vi "Export_Clipboard.vi"(7 "Is Copy? (F)":bool, 8 "error in (no error)":errorcluster, 11 "Data in":T1={"Class"={"Ants"=refnum, "Layer"=refnum, "Templates"=refnum, "Icon"=refnum, "Glyph"=refnum, "Settings"=refnum, "Tools"=refnum}, "Ref"={"Add Layer"=refnum, "Remove Layer"=refnum, "Line Text"=[], "Body Text Spec"=refnum, "DNL_Font"=refnum, "glyph path str"=refnum, "templates path str"=refnum, "Arrow Up"=refnum, "Arrow Down"=refnum, "IE VI Ref"=refnum, "Glyphs tree"=refnum, "Templates tree"=refnum, "Layer Icon Text"=refnum, "Layer Template"=refnum, "Clipboard"=refnum, "BW icon in"=refnum, "Color icon in"=refnum, "Layer Clust"=refnum, "Body Text"=refnum, "DNL_Framework Templates"=refnum, "Search Templates"=refnum, "TextMarker"=refnum, "Tab Control"=refnum, "Search Glyphs"=refnum, "Line Color"=refnum, "DNL_Glyphs []"=refnum, "Fill Color"=refnum, "Tools"=refnum, "Glyphs tree"=refnum, "Icon"=refnum, "Preview"=refnum, "Ants"=refnum, "Terminals"=refnum, "menu reference"=refnum, "LayerNames"=[], "GlyphLoadAnimation"=refnum, "TemplateLoadAnimation"=refnum, "refreshGlyphs"=refnum, "refreshTemplates"=refnum}, "Support"={"AntsRect"={"left"=0, "top"=0, "right"=0, "bottom"=0}, "Mouse Move Coords"={"Horizontal"=0, "Vertical"=0}, "Mouse Down Coords"={"Horizontal"=0, "Vertical"=0}, "Temp Coord"={"Horizontal"=0, "Vertical"=0}, "Action"=enum."Default", "Edge Color"=4914962, "Fill Color"=16860, "Mouse Down?"=FALSE, "Draft Mode?"=FALSE, "Temp Icon"=bytes[3102], "CTRL Pressed"=FALSE, "Move Selection?"=FALSE, "AntsRect Orig"={"left"=0, "top"=0, "right"=0, "bottom"=0}, "Text"="", "TM Set?"=FALSE, "Mouse inside icon?"=FALSE, "Tool (old value)"=0, "Pencil Move Color"=0, "Swap Colors?"=FALSE, "Shift pressed?"=FALSE}}) -> (0 "error out":errorcluster, 3 "Data out":T1={"Class"={"Ants"=refnum, "Layer"=refnum, "Templates"=refnum, "Icon"=refnum, "Glyph"=refnum, "Settings"=refnum, "Tools"=refnum}, "Ref"={"Add Layer"=refnum, "Remove Layer"=refnum, "Line Text"=[], "Body Text Spec"=refnum, "DNL_Font"=refnum, "glyph path str"=refnum, "templates path str"=refnum, "Arrow Up"=refnum, "Arrow Down"=refnum, "IE VI Ref"=refnum, "Glyphs tree"=refnum, "Templates tree"=refnum, "Layer Icon Text"=refnum, "Layer Template"=refnum, "Clipboard"=refnum, "BW icon in"=refnum, "Color icon in"=refnum, "Layer Clust"=refnum, "Body Text"=refnum, "DNL_Framework Templates"=refnum, "Search Templates"=refnum, "TextMarker"=refnum, "Tab Control"=refnum, "Search Glyphs"=refnum, "Line Color"=refnum, "DNL_Glyphs []"=refnum, "Fill Color"=refnum, "Tools"=refnum, "Glyphs tree"=refnum, "Icon"=refnum, "Preview"=refnum, "Ants"=refnum, "Terminals"=refnum, "menu reference"=refnum, "LayerNames"=[], "GlyphLoadAnimation"=refnum, "TemplateLoadAnimation"=refnum, "refreshGlyphs"=refnum, "refreshTemplates"=refnum}, "Support"={"AntsRect"={"left"=0, "top"=0, "right"=0, "bottom"=0}, "Mouse Move Coords"={"Horizontal"=0, "Vertical"=0}, "Mouse Down Coords"={"Horizontal"=0, "Vertical"=0}, "Temp Coord"={"Horizontal"=0, "Vertical"=0}, "Action"=enum."Default", "Edge Color"=4914962, "Fill Color"=16860, "Mouse Down?"=FALSE, "Draft Mode?"=FALSE, "Temp Icon"=bytes[3102], "CTRL Pressed"=FALSE, "Move Selection?"=FALSE, "AntsRect Orig"={"left"=0, "top"=0, "right"=0, "bottom"=0}, "Text"="", "TM Set?"=FALSE, "Mouse inside icon?"=FALSE, "Tool (old value)"=0, "Pencil Move Color"=0, "Swap Colors?"=FALSE, "Shift pressed?"=FALSE}})   [LabVIEW 2021]
uses:
  Controls/IE Data.ctl
  Class/Ants/Ants.lvclass
  Class/FakedArray/FakedArray.lvclass
  vi.lib/LabVIEW Icon API/lv_icon/Classes/Icon/Icon.lvclass
  Class/Icon Library/Glyph.lvclass
  Class/Settings/Settings.lvclass
  Class/Tools/Tools Paint.lvclass
  Controls/IE Classes.ctl
  Controls/References Cluster.ctl
  Controls/SupportClass.ctl
  <vilib>/Utility/miscctls.llb/LVPoint32TypeDef.ctl
  Controls/SupportClass_Action.ctl
  vi.lib/LabVIEW Icon API/lv_icon/Controls/IEColor.ctl
  vi.lib/LabVIEW Icon API/lv_icon/Classes/Icon Framework/Icon Framework.lvclass
  C:/projects/labview-icon-editor/source/vi.lib/LabVIEW Icon API/lv_icon/Classes/Layer/Layer.lvclass
  vi.lib/LabVIEW Icon API/lv_icon/lv_icon.lvlib
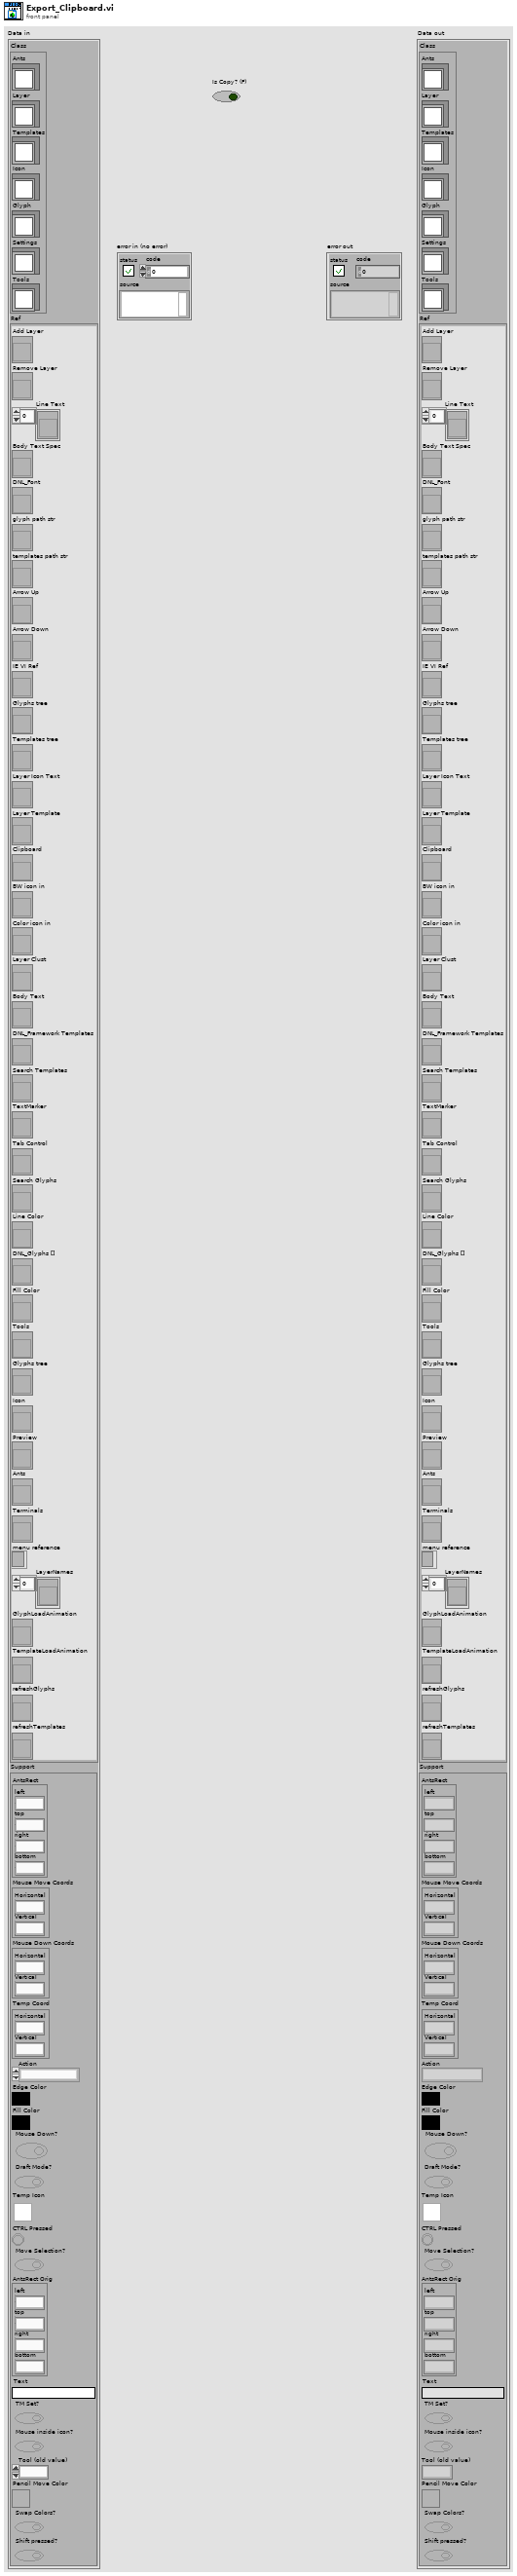
[diagram p1: front panel]
types:
  T1 = typedef "IE Data.ctl" = cluster{"Class":T2, "Ref":T3, "Support":T4}
  T2 = typedef "IE Classes.ctl" = cluster{"Ants":refnum<class "Ants.lvclass">, "Layer":refnum<class "FakedArray.lvclass">, "Templates":refnum<class "FakedArray.lvclass">, "Icon":refnum<class "Icon.lvclass">, "Glyph":refnum<class "Glyph.lvclass">, "Settings":refnum<class "Settings.lvclass">, "Tools":refnum<class "Tools Paint.lvclass">}
  T3 = typedef "References Cluster.ctl" = cluster{"Add Layer":refnum<vi>, "Remove Layer":refnum<vi>, "Line Text":refnum<vi>[], "Body Text Spec":refnum<vi>, "DNL_Font":refnum<vi>, "glyph path str":refnum<vi>, "templates path str":refnum<vi>, "Arrow Up":refnum<vi>, "Arrow Down":refnum<vi>, "IE VI Ref":refnum<vi>, "Glyphs tree":refnum<vi>, "Templates tree":refnum<vi>, "Layer Icon Text":refnum<vi>, "Layer Template":refnum<vi>, "Clipboard":refnum<vi>, "BW icon in":refnum<vi>, "Color icon in":refnum<vi>, "Layer Clust":refnum<vi>, "Body Text":refnum<vi>, "DNL_Framework Templates":refnum<vi>, "Search Templates":refnum<vi>, "TextMarker":refnum<vi>, "Tab Control":refnum<vi>, "Search Glyphs":refnum<vi>, "Line Color":refnum<vi>, "DNL_Glyphs []":refnum<vi>, "Fill Color":refnum<vi>, "Tools":refnum<vi>, "Glyphs tree":refnum<vi>, "Icon":refnum<vi>, "Preview":refnum<vi>, "Ants":refnum<vi>, "Terminals":refnum<vi>, "menu reference":refnum<k9>, "LayerNames":refnum<vi>[], "GlyphLoadAnimation":refnum<vi>, "TemplateLoadAnimation":refnum<vi>, "refreshGlyphs":refnum<vi>, "refreshTemplates":refnum<vi>}
  T4 = typedef "SupportClass.ctl" = cluster{"AntsRect":cluster{"left":i16, "top":i16, "right":i16, "bottom":i16}, "Mouse Move Coords":T5, "Mouse Down Coords":T5, "Temp Coord":T5, "Action":T6, "Edge Color":T7, "Fill Color":T7, "Mouse Down?":bool, "Draft Mode?":bool, "Temp Icon":picture, "CTRL Pressed":bool, "Move Selection?":bool, "AntsRect Orig":cluster{"left":i16, "top":i16, "right":i16, "bottom":i16}, "Text":string, "TM Set?":bool, "Mouse inside icon?":bool, "Tool (old value)":u32, "Pencil Move Color":u32, "Swap Colors?":bool, "Shift pressed?":bool}
  T5 = typedef "LVPoint32TypeDef.ctl" = cluster{"Horizontal":i32, "Vertical":i32}
  T6 = typedef "SupportClass_Action.ctl" = enum16{"Default", "Move Selection", "Glyph Library", "Tool"}
  T7 = typedef "IEColor.ctl" = u32
  T8 = cluster{"left":i16, "top":i16, "right":i16, "bottom":i16}
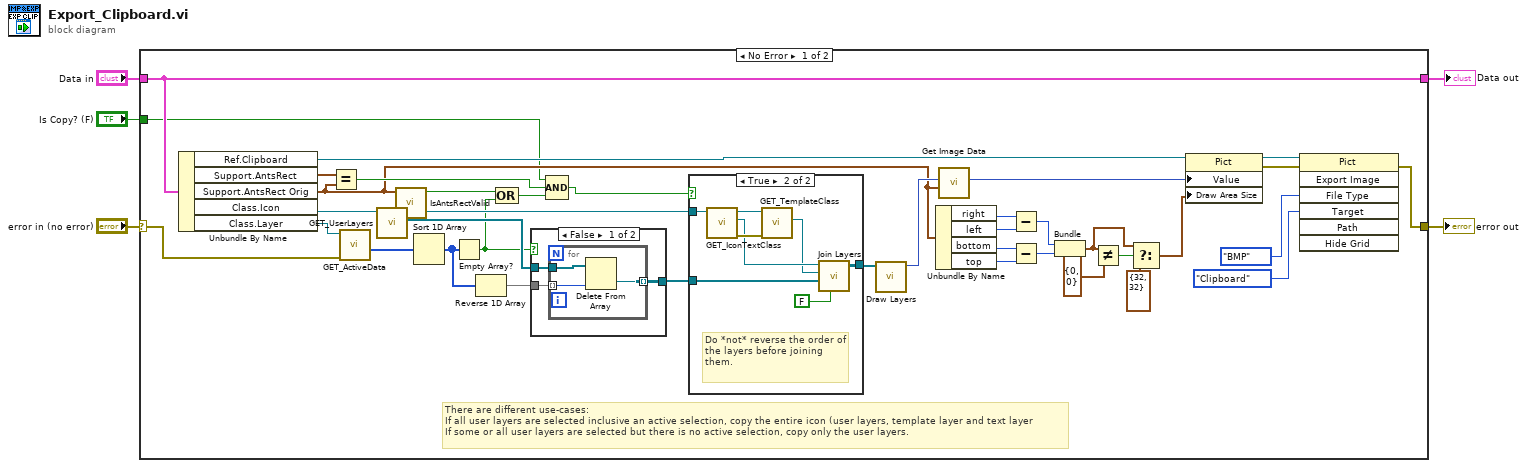
[diagram p0: block diagram]
diagram:
  n1 = case shown="No Error" "error in (no error)" {
    selector: "error in (no error)" -> [w30 w61]
    tunnel: [w34 w61] -> w4
    tunnel: [w16 w60] -> w3
    tunnel: "Data in" -> [w16 w60]
    tunnel: "Is Copy? (F)" -> [w6 _]
    frame No Error {
      # "There are different use-cases:\nIf all user layers are selected inclusive an active selection, copy the entire icon (user layers, template layer and text layer\nIf some or all user layers are selected but there is no active selection, copy only the user layers."
      n2 = Unbundle By Name(w16) -> ("Ref.Clipboard"=w31:refnum<vi>, "Support.AntsRect"=w9:T8, "Support.AntsRect Orig"=w8:T8, "Class.Icon"=w14:refnum<class "Icon.lvclass">, "Class.Layer"=w15:refnum<class "FakedArray.lvclass">)
      n3 = Equal?(x=w9, y=w8) -> (x = y?=w11:bool)
      n4 = call-dynamic "GET_ActiveData.vi"("error in (no error)"=w30, "FakedArray in"=w15) -> ("Active Data []"=w27:i32[])  [unwired: 9 out]
      n5 = call-dynamic "GET_UserLayers.vi"("Icon.lvclass in"=w14) -> ("All Layers"=w28:refnum<class "Layer.lvclass">[], "Icon.lvclass out"=w19:refnum<class "Icon.lvclass">)  [unwired: 1 in, 8 out]
      n6 = call "IsAntsRectValid.vi"("AntsRect"=w8) -> ("Valid?"=w17:bool)  [unwired: 10 out]
      n7 = Sort 1D Array(array=w27) -> (sorted array=w26:i32[])
      n8 = Empty Array?(array=w26) -> (empty?=w7:bool)
      n9 = Reverse 1D Array(array=w26) -> (reversed array=w25:i32[])
      n10 = Compound Arithmetic op=OR(w17, w7) -> (w12:bool)
      n11 = case shown="False" w7 {
        tunnel: w28 -> [w55 w59]
        tunnel: [w54 w59] -> w18
        tunnel: w25 -> [w53 _]
        frame False {
          n12 = for {
            tunnel: w55 -> [w57]
            tunnel: w53 -> [w58] mode=indexing
            tunnel: [w56] -> w54 mode=indexing
            n13 = Delete From Array(array=w57, index=w58) -> (deleted portion=w56:refnum<class "Layer.lvclass">)  [unwired: 1 in, 1 out]
          }
        }
        frame True {
        }
      }
      n14 = Compound Arithmetic op=AND(w6, w11, w12) -> (w10:bool)
      n15 = case shown="True" w10 {
        tunnel: w19 -> [_ w50]
        tunnel: [w44 w49] -> w13
        tunnel: w18 -> [w44 w46]
        frame False {
        }
        frame True {
          # "Do *not* reverse the order of the layers before joining them."
          n16 = call-dynamic "GET_IconTextClass.vi"("Icon.lvclass in"=w50) -> ("error out"=w52:errorcluster, "Icon Framework.lvclass"=w48:refnum<class "Icon Framework.lvclass">, "Icon.lvclass out"=w51:refnum<class "Icon.lvclass">)  [unwired: 1 in, 7 out]
          n17 = call-dynamic "GET_TemplateClass.vi"("error in (no error)"=w52, "Icon.lvclass in"=w51) -> ("Icon Framework.lvclass"=w47:refnum<class "Icon Framework.lvclass">)  [unwired: 9 out]
          n18 = call "Join Layers.vi"("Rotate? (T)"=FALSE, "User Layers"=w46, "Template"=w47, "Icon Text"=w48) -> ("Layer out"=w49:refnum<class "Layer.lvclass">[])  [unwired: 2 in, 5 out]
        }
      }
      n19 = call "Draw Layers.vi"("Layers"=w13) -> ("Picture"=w29:picture)  [unwired: 4 in, 6 out]
      n20 = Unbundle By Name(w8) -> ("right"=w43:i16, "left"=w42:i16, "bottom"=w41:i16, "top"=w40:i16)
      n21 = call "Get Image Data.vi"("subset rect"=w8, "Pic In"=w29) -> ("Pic Out"=w32:picture)  [unwired: 1 in, 8 out]
      n22 = Subtract(x=w43, y=w42) -> (x-y=w38:i16)
      n23 = Subtract(x=w41, y=w40) -> (x-y=w39:i16)
      n24 = Bundle(w38, w39) -> (w22:cluster{i16, i16})  [unwired: 1 out]
      n25 = Not Equal?(x=w22, y=cluster{i16, i16} {0, 0}) -> (x != y?=w23:bool)
      n26 = Select(t=w22, s=w23, f=cluster{i16, i16} {32, 32}) -> (s? t:f=w20:cluster{i16, i16})
      n27 = property on="Property Node" class="Pict"(reference=w31, "Value"=w32, "Draw Area Size"=w20) -> (reference out=w33:refnum<vi>, error out=w37:errorcluster)  [unwired: 1 in]
      n28 = invoke on="Invoke Node" class="Pict" method="Export Image"(reference=w33, error in=w37, "File Type"=enum32{"BMP", "EPS", "EMF", "PICT"}."BMP", "Target"=enum32{"File", "Clipboard"}."Clipboard") -> (error out=w34:errorcluster)  [unwired: 3 in, 6 out]
    }
    frame Error {
    }
  }
  "error out" <- w4
  "Data out" <- w3
